vi "Preview.vi"(6 "Local Data":T1, 7 "UI Refs":T9, 8 "error in (no error)":errorcluster, 9 "Coords":T8) -> (0 "error out":errorcluster, 4 "Local Data out":T1)   [LabVIEW 2024]
uses:
  Controls/RVHR - UI Refs.ctl
  <vilib>/Utility/miscctls.llb/LVPoint32TypeDef.ctl
  Controls/RVHR - Local Data.ctl
  Controls/Test Cluster.ctl
  Controls/Excluded Information.ctl
  Controls/Language.ctl
  Controls/Device_Type.ctl
  <vilib>/Utility/miscctls.llb/LVRectTypeDef.ctl
  <vilib>/Utility/miscctls.llb/LVBoundsTypeDef.ctl
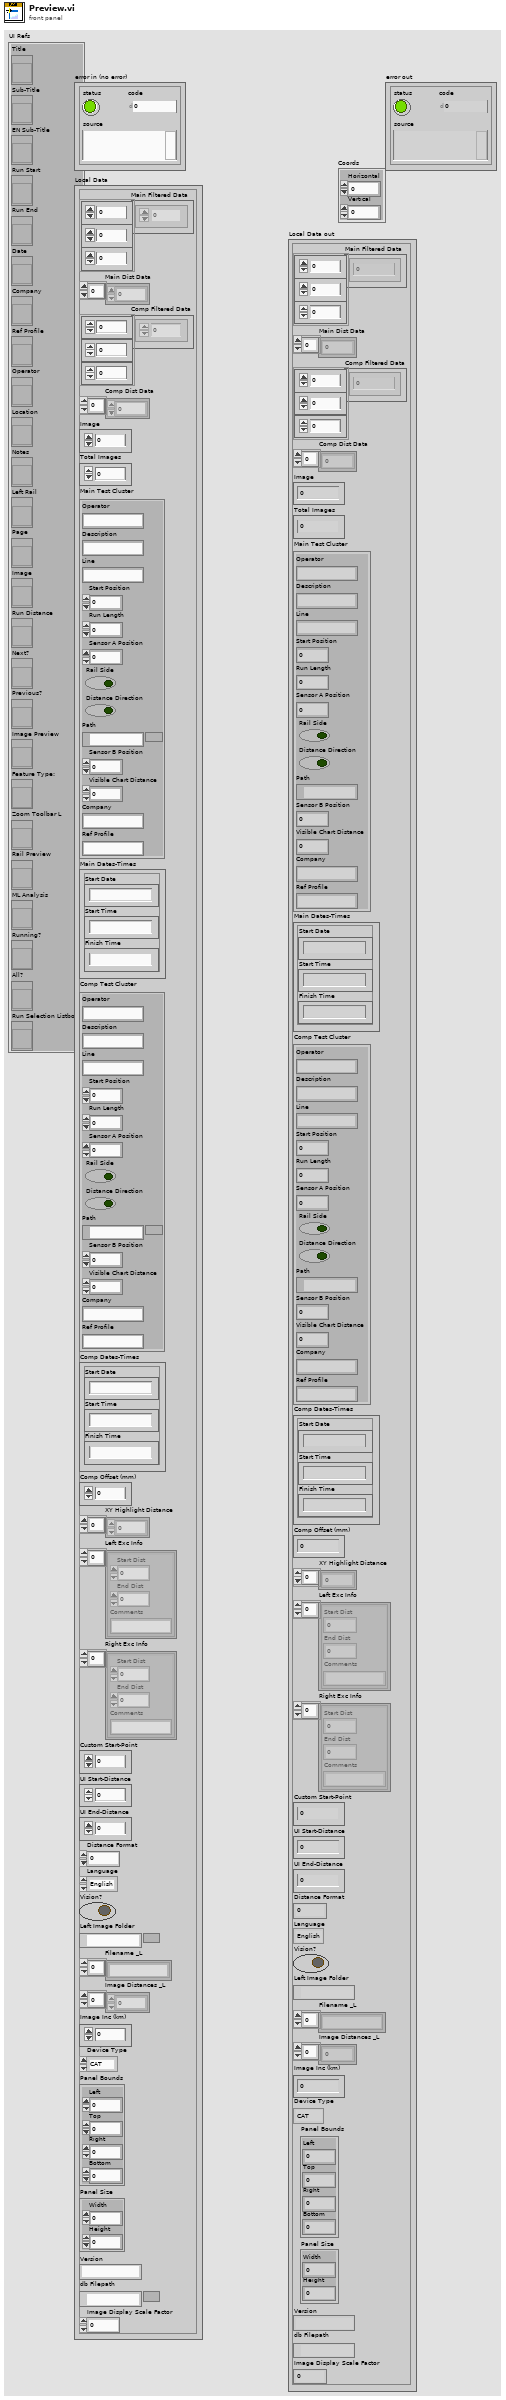
[diagram p1: front panel]
types:
  T1 = typedef "RVHR - Local Data.ctl" = cluster{"Main Filtered Data":dbl[][][], "Main Dist Data":dbl[], "Comp Filtered Data":dbl[][][], "Comp Dist Data":dbl[], "Image":u16, "Total Images":u16, "Main Test Cluster":T2, "Main Dates-Times":cluster{"Start Date":string, "Start Time":string, "Finish Time":string}, "Comp Test Cluster":T2, "Comp Dates-Times":cluster{"Start Date":string, "Start Time":string, "Finish Time":string}, "Comp Offset (mm)":i64, "XY Highlight Distance":dbl[], "Left Exc Info":T3[], "Right Exc Info":T3[], "Custom Start-Point":dbl, "UI Start-Distance":dbl, "UI End-Distance":dbl, "Distance Format":u8, "Language":T4, "Vision?":bool, "Left Image Folder":path, "Filename _L":string[], "Image Distances _L":dbl[], "Image Inc (km)":dbl, "Device Type":T5, "Panel Bounds":T6, "Panel Size":T7, "Version":string, "db Filepath":path, "Image Display Scale Factor":dbl}
  T2 = typedef "Test Cluster.ctl" = cluster{"Operator":string, "Description":string, "Line":string, "Start Position":dbl, "Run Length":dbl, "Sensor A Position":dbl, "Rail Side":bool, "Distance Direction":bool, "Path":path, "Sensor B Position":dbl, "Visible Chart Distance":dbl, "Company":string, "Ref Profile":string}
  T3 = typedef "Excluded Information.ctl" = cluster{"Start Dist":dbl, "End Dist":dbl, "Comments":string}
  T4 = typedef "Language.ctl" = enum16{"English", "Chinese", "German"}
  T5 = typedef "Device_Type.ctl" = enum16{"CAT", "Bi-CAT", "YRCA", "RCA", "RV-HR", "TV-HR"}
  T6 = typedef "LVRectTypeDef.ctl" = cluster{"Left":i16, "Top":i16, "Right":i16, "Bottom":i16}
  T7 = typedef "LVBoundsTypeDef.ctl" = cluster{"Width":u32, "Height":u32}
  T8 = typedef "LVPoint32TypeDef.ctl" = cluster{"Horizontal":i32, "Vertical":i32}
  T9 = typedef "RVHR - UI Refs.ctl" = cluster{"Title":refnum<vi>, "Sub-Title":refnum<vi>, "EN Sub-Title":refnum<vi>, "Run Start":refnum<vi>, "Run End":refnum<vi>, "Date":refnum<vi>, "Company":refnum<vi>, "Ref Profile":refnum<vi>, "Operator":refnum<vi>, "Location":refnum<vi>, "Notes":refnum<vi>, "Left Rail":refnum<vi>, "Page":refnum<vi>, "Image":refnum<vi>, "Run Distance":refnum<vi>, "Next?":refnum<vi>, "Previous?":refnum<vi>, "Image Preview":refnum<vi>, "Feature Type:":refnum<vi>, "Zoom Toolbar L":refnum<vi>, "Rail Preview":refnum<vi>, "ML Analysis":refnum<vi>, "Running?":refnum<vi>, "All?":refnum<vi>, "Run Selection Listbox":refnum<vi>}
  T10 = typedef "LVMouseTypeDef.ctl" = cluster{"Mouse Position":cluster{"X":i32, "Y":i32}, "Mouse Modifiers":cluster{"Button Down":bool, "Shift Mod":bool, "Menu Mod":bool, "Option Mod":bool}}
  T11 = typedef "imagedata.ctl" = cluster{"image type":i32, "image depth":i32, "image":u8[], "mask":u8[], "colors":u32[], "Rectangle":cluster{"left":i16, "top":i16, "right":i16, "bottom":i16}}
  T12 = cluster{"left":i16, "top":i16, "right":i16, "bottom":i16}
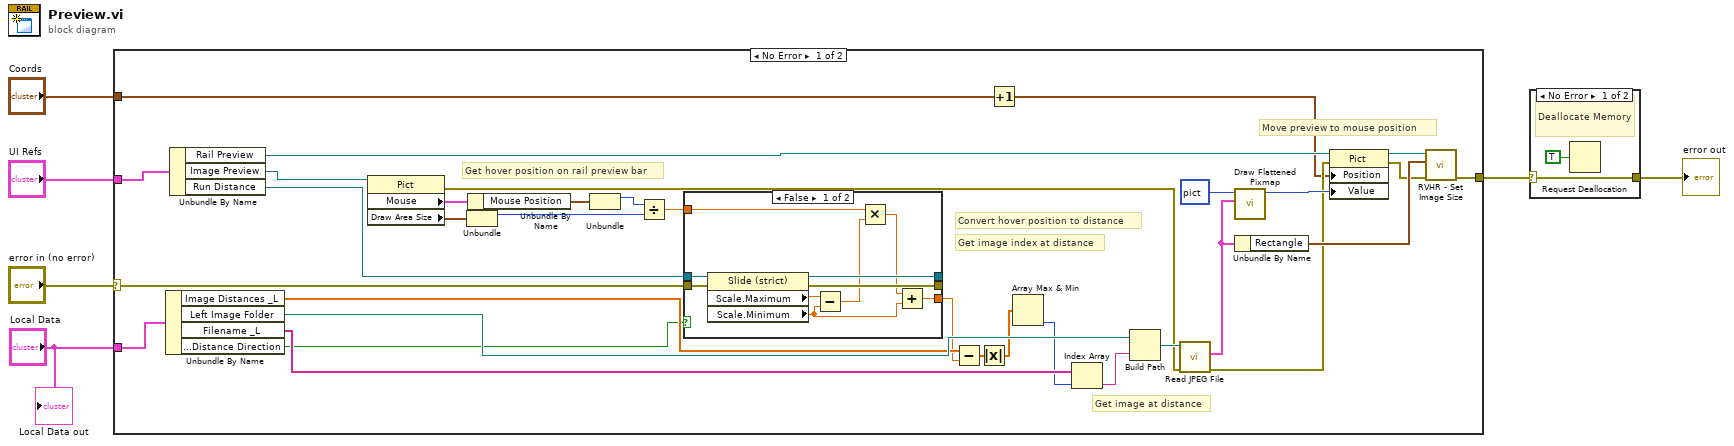
[diagram p0: block diagram]
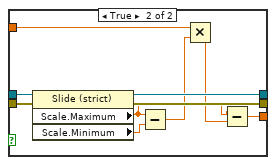
[diagram p3: hidden frame]
diagram:
  n1 = case shown="No Error" "error in (no error)" {
    selector: "error in (no error)" -> [w13 w60]
    tunnel: "UI Refs" -> [w39 _]
    tunnel: "Coords" -> [w15 _]
    tunnel: "Local Data" -> [w37 _]
    tunnel: [w17 w60] -> w2
    frame No Error {
      # "Move preview to mouse position"
      # "Get image at distance"
      # "Get image index at distance"
      # "Convert hover position to distance"
      # "Get hover position on rail preview bar"
      n2 = Unbundle By Name(w37) -> ("Image Distances _L"=w27:dbl[], "Left Image Folder"=w36:path, "Filename _L"=w35:string[], "Main Test Cluster.Distance Direction"=w10:bool)
      n3 = Unbundle By Name(w39) -> ("Rail Preview"=w23:refnum<vi>, "Image Preview"=w38:refnum<vi>, "Run Distance"=w12:refnum<vi>)
      n4 = property class="Pict"(reference=w38) -> (error out=w16:errorcluster, "Mouse"=w31:T10, "Draw Area Size"=w32:T7)  [unwired: 1 in, 1 out]
      n5 = Unbundle(w32) -> ("Width"=w29:u32)  [unwired: 1 out]
      n6 = Unbundle By Name(w31) -> ("Mouse Position"=w30:cluster{"X":i32, "Y":i32})
      n7 = Unbundle(w30) -> ("X"=w28:i32)  [unwired: 1 out]
      n8 = Divide(x=w28, y=w29) -> (x/y=w11:dbl)
      n9 = case shown="False" w10 {
        tunnel: [w49 w59] -> _
        tunnel: w12 -> [w47 w58]
        tunnel: [w46 w57] -> _
        tunnel: [w42 w55] -> w8
        tunnel: w13 -> [w41 w54]
        tunnel: w11 -> [w40 w53]
        frame False {
          n10 = property class="Slide (strict)"(reference=w47, error in=w41) -> (reference out=w49:refnum<vi>, error out=w46:errorcluster, "Scale.Maximum"=w48:dbl, "Scale.Minimum"=w43:dbl)
          n11 = Subtract(x=w48, y=w43) -> (x-y=w45:dbl)
          n12 = Multiply(x=w40, y=w45) -> (x*y=w44:dbl)
          n13 = Add(x=w44, y=w43) -> (x+y=w42:dbl)
        }
        frame True {
          n14 = property class="Slide (strict)"(reference=w58, error in=w54) -> (reference out=w59:refnum<vi>, error out=w57:errorcluster, "Scale.Maximum"=w52:dbl, "Scale.Minimum"=w51:dbl)
          n15 = Subtract(x=w52, y=w51) -> (x-y=w56:dbl)
          n16 = Multiply(x=w53, y=w56) -> (x*y=w50:dbl)
          n17 = Subtract(x=w52, y=w50) -> (x-y=w55:dbl)
        }
      }
      n18 = Subtract(x=w27, y=w8) -> (x-y=w9:dbl[])
      n19 = Absolute Value(x=w9) -> (abs(x)=w7:dbl[])
      n20 = Increment(x=w15) -> (x+1=w14:T8)
      n21 = Array Max & Min(array=w7) -> (min index (indices)=w26:i32)  [unwired: 3 out]
      n22 = Index Array(array=w35, index=w26) -> (element=w34:string)
      n23 = Build Path(base path=w36, name or relative path=w34) -> (appended path=w33:path)
      n24 = call <vilib>:"Read JPEG File.vi"("error in (no error)"=w16, "path to JPEG file"=w33) -> ("error out"=w18:errorcluster, "image data"=w25:T11)  [unwired: 7 in, 1 out]
      n25 = call <vilib>:"Draw Flattened Pixmap.vi"("image data"=w25, "picture"=picture data[5B]) -> ("new picture"=w21:picture)  [unwired: 7 in]
      n26 = Unbundle By Name(w25) -> ("Rectangle"=w24:T12)
      n27 = property class="Pict"(reference=w23, error in=w18, "Position"=w14, "Value"=w21) -> (reference out=w20:refnum<vi>, error out=w19:errorcluster)
      n28 = call "RVHR - Set Image Size.vi"("error in (no error)"=w19, "Rectangle"=w24, "Image_L"=w20) -> ("error out"=w17:errorcluster)  [unwired: 8 in]
    }
    frame Error {
    }
  }
  n29 = case shown="No Error" w2 {
    selector: w2 -> [w61 w63]
    tunnel: [w61 w63] -> w1
    frame No Error {
      # "Deallocate Memory"
      n30 = Request Deallocation(TRUE ("flag")) -> ()
    }
    frame Error {
    }
  }
  "error out" <- w1
  "Local Data out" <- "Local Data"
